vi "T17.vi"(2 "Parametry Ziemi":T1={"a - półoś duża"=6378137.0, "b - półoś mała"=6356752.3141999999998} {"b - półoś mała" format="%_20f"; "a - półoś duża" format="%_20g"}, 3 "fi'":ext) -> (7 "T17":ext)   [LabVIEW 2012, in "Biblioteka moduł map v3.lvlib" / "Konwersja wsp.lvlib" / "UTM.lvlib" / "Konwersja z UTM na wsp geograficzne.lvlib"]
uses:
  Konwersja z UTM na wsp geograficzne.lvlib
  UTM.lvlib
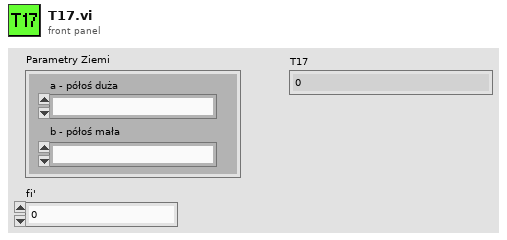
[diagram p1: front panel]
types:
  T1 = cluster{"a - półoś duża":ext, "b - półoś mała":ext}
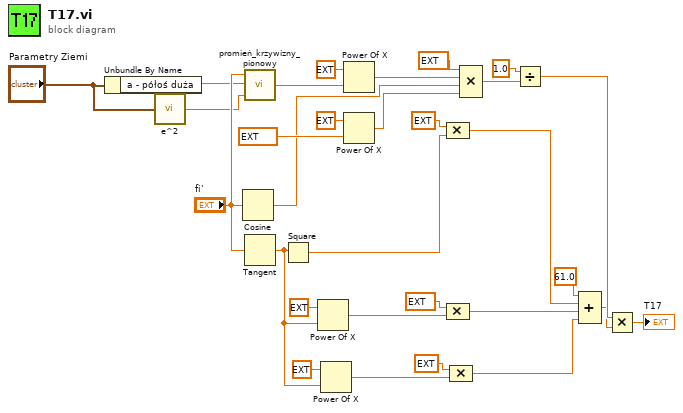
[diagram p0: block diagram]
diagram:
  n1 = Unbundle By Name("Parametry Ziemi") -> ("a - półoś duża"=w3:ext)
  n2 = call "e^2.vi"("Parametry Ziemi"="Parametry Ziemi") -> ("e^2"=w1:ext)  [unwired: 4 in]
  n3 = Cosine(x="fi'") -> (cos(x)=w14:ext)
  n4 = call "promień_krzywizny_pionowy.vi"("e^2"=w1, "a"=w3, "fi[rad]"="fi'") -> ("Promien krzywizny równoleżnika"=w28:ext)  [unwired: 2 in]
  n5 = Tangent(1:"fi'") -> (0:w10:ext)
  n6 = Square(x=w10) -> (x^2=w11:ext)
  n7 = Power Of X(1:w10, 2:ext 4.0 ("y")) -> (0:w5:ext)
  n8 = Power Of X(1:w10, 2:ext 6.0 ("y")) -> (0:w4:ext)
  n9 = Power Of X(1:w28, 2:ext 7.0 ("y")) -> (0:w26:ext)
  n10 = Power Of X(1:ext 0.9996 ("k0"), 2:ext 7.0 ("y")) -> (0:w22:ext)
  n11 = Compound Arithmetic op=MULTIPLY(ext 662.0 ("value"), w11) -> (w16:ext)
  n12 = Compound Arithmetic op=MULTIPLY(ext 1320.0 ("value"), w5) -> (w7:ext)
  n13 = Compound Arithmetic op=MULTIPLY(ext 720.0 ("value"), w4) -> (w6:ext)
  n14 = Compound Arithmetic op=MULTIPLY(ext 5040.0 ("value"), w26, w14, w22) -> (w29:ext)
  n15 = Divide(x=1.0, y=w29) -> (x/y=w21:ext)
  n16 = Compound Arithmetic op=ADD(61.0 ("value"), w16, w7, w6) -> (w20:ext)
  n17 = Multiply(x=w21, y=w20) -> (x*y=→"T17":ext)
